vi "Make_RDDF_KBS.vi"() -> ()   [LabVIEW 2020]
uses:
  <vilib>/Utility/file.llb/Read Delimited Spreadsheet (DBL).vi
  <vilib>/Utility/file.llb/Write Delimited Spreadsheet (DBL).vi
panel:
  out "Y(long)":dbl format="%#_12g"
  out "X(lat)":dbl format="%#_12g"
  in  "stop":bool
  in  "file path (dialog if empty)":path caption="파일 경로(비었을 경우 대화 상자 창)"
  in  "dist.":dbl=0.2
  in  "?":bool
  out "XY 그래프":cluster{dbl[], dbl[]}[](graph)
  in  "File_Name(User):":string
  out "File_Name(Save):":string
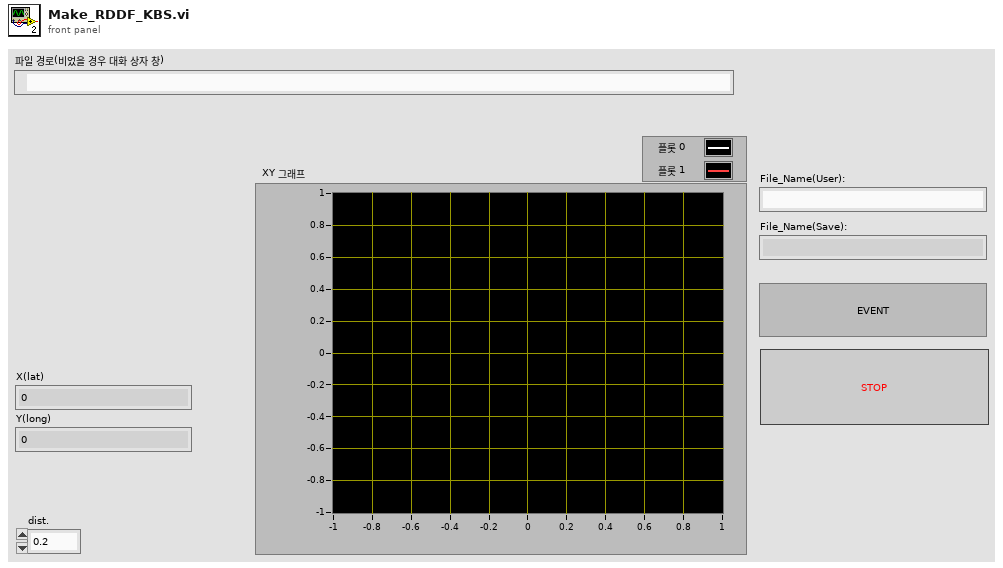
[diagram p1: front panel]
types:
  T1 = cluster{"X(lat)":dbl, "Y(long)":dbl, "Heading_T":dbl, "Heading_M":dbl, "GPS_SPD(kph)":dbl}
  T2 = enum16{"open", "replace", "create", "open or create", "replace or create", "replace or create with confirmation"}
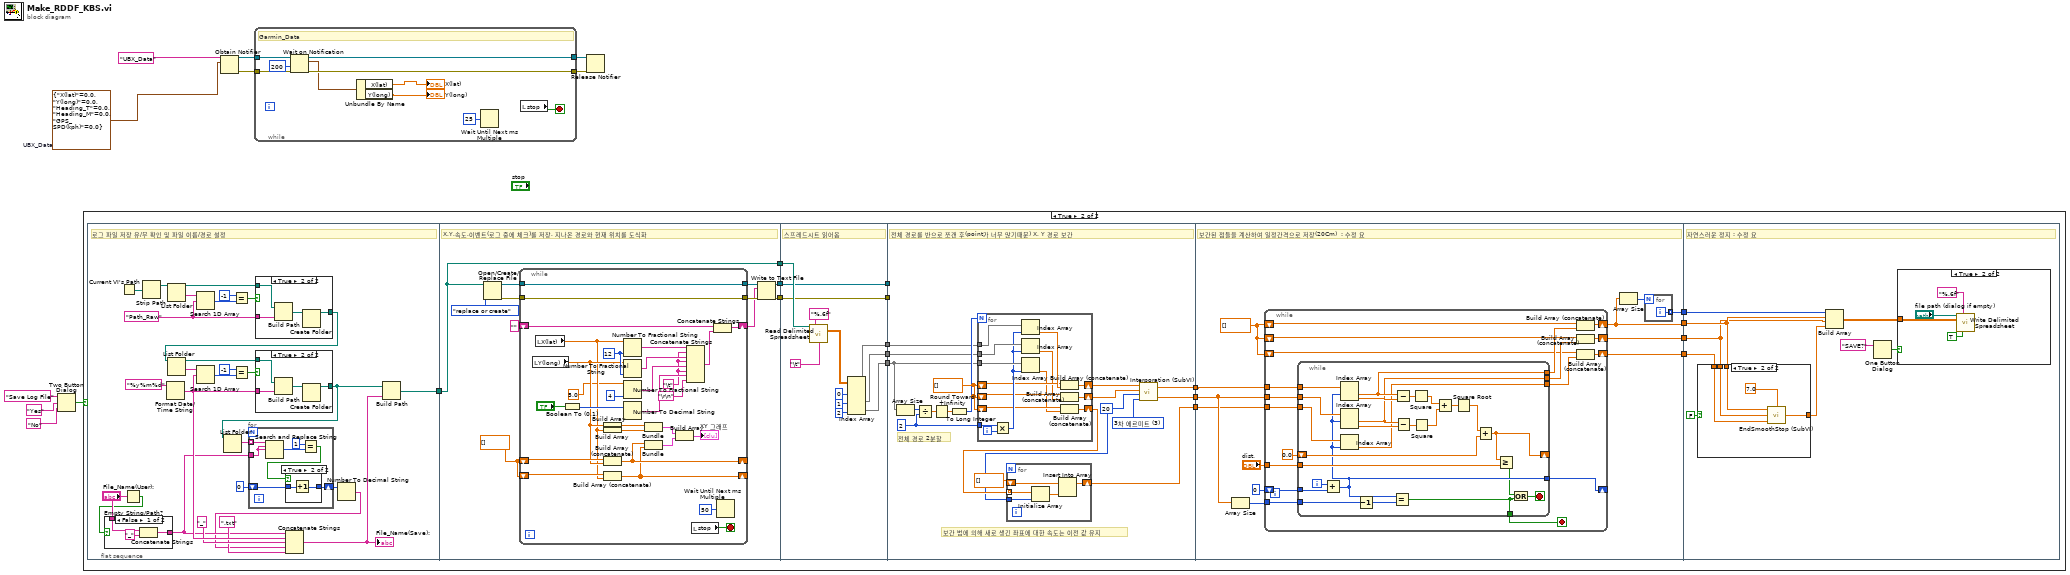
[diagram p0: block diagram]
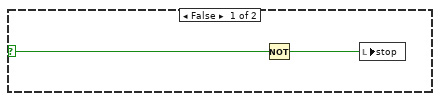
[diagram p2: hidden frame]
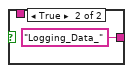
[diagram p3: hidden frame]
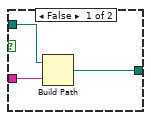
[diagram p5: hidden frame]
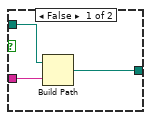
[diagram p6: hidden frame]
diagram:
  w1 = T1 {"X(lat)"=0.0, "Y(long)"=0.0, "Heading_T"=0.0, "Heading_M"=0.0, "GPS_SPD(kph)"=0.0}  # UBX_Data
  n1 = Two Button Dialog(message="Save Log File" ("메시지"), 1:"No" ("거짓 버튼 이름(\"취소\")"), 2:"Yes" ("참 버튼 이름(\"확인\")")) -> (T button?=w7:bool)
  n2 = case shown="True" w7 {
    selector: w7 -> [w12 _]
    frame False {
      n3 = Not(x=w12) -> (.not. x?=w11:bool)
      n4 = local write "stop"(w11) -> ()
    }
    frame True {
      n5 = flat-sequence {
        tunnel: [w56] -> w28
        tunnel: w28 -> [w88]
        tunnel: [w88] -> w27
        tunnel: [w87] -> w26
        tunnel: [w86] -> w25
        tunnel: w27 -> [w136]
        tunnel: w26 -> [w132]
        tunnel: w25 -> [w133]
        tunnel: [w133] -> w23
        tunnel: [w132] -> w22
        tunnel: [w125] -> w21
        tunnel: [w126] -> w20
        tunnel: [w130] -> w19
        tunnel: [w143] -> w24
        tunnel: w23 -> [_]
        tunnel: w22 -> [_]
        tunnel: w21 -> [w147]
        tunnel: w20 -> [w148]
        tunnel: w19 -> [w149]
        tunnel: [w138] -> w18
        tunnel: [w137] -> w17
        tunnel: w24 -> [w179]
        tunnel: w18 -> [w181]
        tunnel: w17 -> [w180]
        tunnel: [w178] -> w16
        tunnel: [w177] -> w15
        tunnel: [w176] -> w14
        tunnel: [w175] -> w13
        tunnel: w16 -> [w236]
        tunnel: w15 -> [w235]
        tunnel: w14 -> [w231]
        tunnel: w13 -> [w232]
        frame #0 {
          w51 = "Path_Raw" ("원소")
          # "로그 파일 저장 유/무 확인 및 파일 이름/경로 설정"
          n6 = Current VI's Path() -> (path=w55:path)
          n7 = Empty String/Path?(string/path="File_Name(User):") -> (empty?=w31:bool)
          n8 = case shown="False" w31 {
            tunnel: [w58 "Logging_Data_"] -> w35
            tunnel: "File_Name(User):" -> [w57 _]
            frame False {
              n9 = Concatenate Strings(w57, "_" ("문자열")) -> (w58:string)
            }
            frame True {
            }
          }
          n10 = Strip Path(path=w55) -> (stripped path=w54:path)  [unwired: 1 out]
          n11 = Format Date/Time String(time format string (%c)="%y%m%d" ("시간 포맷 문자열 (%c)")) -> (date/time string=w38:string)  [unwired: 2 in]
          n12 = List Folder(path=w54) -> (path out=w53:path, folder names=w50:string[])  [unwired: 3 in, 2 out]
          n13 = Search 1D Array(1D array=w50, element=w51) -> (index of element=w49:i32)  [unwired: 1 in]
          n14 = Equal?(x=-1 ("y"), y=w49) -> (x = y?=w52:bool)
          n15 = case shown="True" w52 {
            tunnel: w53 -> [w78 w83]
            tunnel: w51 -> [w79 w82]
            tunnel: [w80 w81] -> w41
            frame False {
              n16 = Build Path(base path=w78, name or relative path=w79) -> (appended path=w80:path)
            }
            frame True {
              n17 = Build Path(base path=w83, name or relative path=w82) -> (appended path=w84:path)
              n18 = Create Folder(path (use dialog)=w84) -> (created path=w81:path)  [unwired: 2 in, 2 out]
            }
          }
          n19 = List Folder(path=w41) -> (path out=w42:path, folder names=w44:string[])  [unwired: 3 in, 2 out]
          n20 = Search 1D Array(1D array=w44, element=w38) -> (index of element=w45:i32)  [unwired: 1 in]
          n21 = Equal?(x=-1 ("y"), y=w45) -> (x = y?=w43:bool)
          n22 = case shown="True" w43 {
            tunnel: w42 -> [w71 w76]
            tunnel: w38 -> [w72 w75]
            tunnel: [w73 w74] -> w30
            frame False {
              n23 = Build Path(base path=w71, name or relative path=w72) -> (appended path=w73:path)
            }
            frame True {
              n24 = Build Path(base path=w76, name or relative path=w75) -> (appended path=w77:path)
              n25 = Create Folder(path (use dialog)=w77) -> (created path=w74:path)  [unwired: 2 in, 2 out]
            }
          }
          n26 = List Folder(path=w30) -> (filenames=w40:string[])  [unwired: 3 in, 3 out]
          n27 = for {
            tunnel: w40 -> [w67] mode=indexing
            shift-right: [w62] -> w34
            shift-left: 0 -> [w63]
            tunnel: w35 -> [w61]
            n28 = Search and Replace String(input string=w67, search string=w61, replace string=w61) -> (number of replacements=w65:i32)  [unwired: 5 in, 3 out]
            n29 = Equal?(x=1, y=w65) -> (x = y?=w64:bool)
            n30 = case shown="True" w64 {
              tunnel: w63 -> [w68 w70]
              tunnel: [w68 w69] -> w62
              frame False {
              }
              frame True {
                n31 = Increment(x=w70) -> (x+1=w69:i32)
              }
            }
          }
          n32 = Number To Decimal String(number=w34) -> (decimal integer string=w33:string)  [unwired: 1 in]
          n33 = Concatenate Strings(w35, w38, "_" ("문자열"), w33, ".txt" ("문자열")) -> (w29:string)
          "File_Name(Save):" <- w29
          n34 = Build Path(base path=w30, name or relative path=w29) -> (appended path=w56:path)
        }
        frame #1 {
          w85 = dbl[] []
          # "X,Y,속도,이벤트(로그 중에 체크)를 저장, 지나온 경로와 현재 위치를 도식화"
          n35 = Open/Create/Replace File(file path (use dialog)=w88, operation (0:open)=T2."replace or create" ("동작(0:open)")) -> (refnum out=w93:refnum<file>, error out=w94:errorcluster)  [unwired: 4 in, 1 out]
          n36 = while {
            tunnel: w94 -> [w119]
            tunnel: w93 -> [w120]
            tunnel: [w120] -> w91
            tunnel: [w119] -> w92
            shift-right: [w104] -> w90
            shift-left: "" -> [w106]
            shift-right: [w100] -> _
            shift-left: w85 -> [w111]
            shift-right: [w99] -> _
            shift-left: w85 -> [w110]
            stop <- w118 stop-if-true
            w113 = "\t"
            w124 = i16 12 ("정밀도(6)")
            n37 = local read "Y(long)"() -> (w98:dbl)
            n38 = local read "X(lat)"() -> (w97:dbl)
            n39 = Boolean To (0,1)(Boolean="?") -> (0, 1=w121:i16)
            n40 = Build Array(w98) -> (w109:dbl[])
            n41 = Build Array(w97) -> (w108:dbl[])
            n42 = Build Array (concatenate)(w111, w98) -> (w100:dbl[])
            n43 = Build Array (concatenate)(w110, w97) -> (w99:dbl[])
            n44 = Number To Fractional String(number=w97, precision (6)=w124) -> (F-format string=w117:string)  [unwired: 2 in]
            n45 = Number To Fractional String(number=w98, precision (6)=w124) -> (F-format string=w116:string)  [unwired: 2 in]
            n46 = Number To Fractional String(number=5.0 ("x vel"), precision (6)=i16 4 ("정밀도(6)")) -> (F-format string=w115:string)  [unwired: 2 in]
            n47 = Number To Decimal String(number=w121) -> (decimal integer string=w114:string)  [unwired: 1 in]
            n48 = Bundle(w109, w108) -> (w101:cluster{dbl[], dbl[]})  [unwired: 1 in]
            n49 = Bundle(w100, w99) -> (w102:cluster{dbl[], dbl[]})  [unwired: 1 in]
            n50 = Build Array(w101, w102) -> (→"XY 그래프":cluster{dbl[], dbl[]}[])
            n51 = Concatenate Strings(w117, w113, w116, w113, w115, w113, w114, "\r\n") -> (w105:string)
            n52 = local read "stop"() -> (w118:bool)
            n53 = Concatenate Strings(w106, w105) -> (w104:string)
            n54 = Wait Until Next ms Multiple(millisecond multiple=u32 50 ("ms 배수")) -> ()  [unwired: 1 out]
          }
          n55 = Write to Text File(file (use dialog)=w91, text=w90, error in=w92) -> (refnum out=w86:refnum<file>, error out=w87:errorcluster)  [unwired: 1 in, 1 out]
        }
        frame #2 {
          # "스프레드시트 읽어옴"
          n56 = call-poly <vilib>:"Read Delimited Spreadsheet.vi"("file path (dialog if empty)"=w136, "format (%.3f)"="%.6f", "delimiter (\\t)"="\t") -> ("all rows"=w131:dbl[][])  [unwired: 7 in, 5 out]
          n57 = Index Array(array=w131, index (col) #1=0 ("비활성화된 인덱스 (열)"), index (col) #2=1 ("인덱스 (열)"), index (col) #3=2 ("인덱스 (열)")) -> (element #1=w130:dbl[], element #2=w126:dbl[], element #3=w125:dbl[])  [unwired: 3 in]
        }
        frame #3 {
          w142 = 3 items=["최근접", "선형", "스플라인", "3차 에르미트", "라그랑지"] ("method")
          w139 = 20 ("Interpolation factor (n)")
          w146 = dbl[] []
          w150 = 2
          # "보간 법에 의해 새로 생긴 좌표에 대한 속도는 이전 값 유지"
          # "전체 경로 2분할"
          # "전체 경로를 반으로 쪼갠 후(point가 너무 많기때문) X, Y 경로 보간"
          n58 = Array Size(array=w147) -> (size(s)=w154:i32)
          n59 = Divide(x=w154, y=w150) -> (x/y=w153:dbl)
          n60 = Round Toward +Infinity(x=w153) -> (ceil(x): smallest int >= x=w152:dbl)
          n61 = To Long Integer(number=w152) -> (32bit integer=w151:i32)
          n62 = for {
            N: w151 -> [_]
            tunnel: w150 -> [w173]
            tunnel: w149 -> [w172]
            tunnel: w148 -> [w171]
            tunnel: w147 -> [w170]
            shift-right: [w166] -> w141
            shift-left: w146 -> [w167]
            shift-right: [w165] -> w140
            shift-left: w146 -> [w163]
            shift-right: [w164] -> w145
            shift-left: w146 -> [w162]
            i -> [w174]
            n63 = Multiply(x=w173, y=w174) -> (x*y=w169:i32)
            n64 = Index Array(array=w172, index=w169) -> (element=w168:dbl)
            n65 = Index Array(array=w171, index=w169) -> (element=w161:dbl)
            n66 = Index Array(array=w170, index=w169) -> (element=w160:dbl)
            n67 = Build Array (concatenate)(w167, w168) -> (w166:dbl[])
            n68 = Build Array (concatenate)(w163, w161) -> (w165:dbl[])
            n69 = Build Array (concatenate)(w162, w160) -> (w164:dbl[])
          }
          n70 = for {
            tunnel: w145 -> [w159] mode=indexing
            tunnel: w139 -> [w158]
            shift-right: [w157] -> w143
            shift-left: dbl[] [] -> [w156]
            n71 = Initialize Array(w159, w158) -> (w155:dbl[])
            n72 = Insert Into Array(array=w156, new element=w155) -> (w157:dbl[])  [unwired: 1 in]
          }
          n73 = call "Interporation (SubVI).vi"("method"=w142, "Sample"=w139, "Y_long"=w140, "X_lat"=w141) -> ("Y_long"=w137:dbl[], "X_lat"=w138:dbl[])
        }
        frame #4 {
          w184 = dbl[] []
          # "보간된 점들을 계산하여 일정간격으로 저장(20Cm)  : 수정 요"
          n74 = Array Size(array=w180) -> (size(s)=w183:i32)
          n75 = while {
            tunnel: "dist." -> [w202]
            tunnel: w181 -> [w205]
            tunnel: w180 -> [w204]
            tunnel: w179 -> [w196]
            shift-right: [w191] -> _
            shift-left: 0 -> [w201]
            shift-right: [w188] -> w175
            shift-left: w184 -> [w197]
            shift-right: [w190] -> w176
            shift-left: w184 -> [w198]
            shift-right: [w189] -> w177
            shift-left: w184 -> [w194]
            tunnel: w183 -> [w193]
            stop <- w192 stop-if-true
            n76 = while {
              tunnel: w205 -> [w230]
              tunnel: w204 -> [w229]
              shift-right: [w219] -> _
              shift-left: 0.0 -> [w220]
              tunnel: w202 -> [w218]
              tunnel: [w210] -> w191
              tunnel: w201 -> [w216]
              tunnel: [w215] -> w200
              tunnel: [w214] -> w199
              tunnel: w196 -> [w213]
              tunnel: [w212] -> w195
              tunnel: w193 -> [w211]
              tunnel: [w207] -> w192
              i -> [w217]
              stop <- w209 stop-if-true
              n77 = Add(x=w217, y=w216) -> (x+y=w210:i32)
              n78 = Index Array(array=w230, index #1=w210) -> (element #1=w215:dbl, element #2=w228:dbl)  [unwired: 1 in]
              n79 = Index Array(array=w229, index #1=w210) -> (element #1=w214:dbl, element #2=w227:dbl)  [unwired: 1 in]
              n80 = Index Array(array=w213, index=w210) -> (element=w212:dbl)
              n81 = Decrement(x=w211) -> (x-1=w206:i32)
              n82 = Equal?(x=w210, y=w206) -> (x = y?=w207:bool)
              n83 = Subtract(x=w215, y=w228) -> (x-y=w226:dbl)
              n84 = Subtract(x=w214, y=w227) -> (x-y=w225:dbl)
              n85 = Square(x=w226) -> (x^2=w224:dbl)
              n86 = Square(x=w225) -> (x^2=w223:dbl)
              n87 = Add(x=w224, y=w223) -> (x+y=w222:dbl)
              n88 = Square Root(x=w222) -> (sqrt(x)=w221:dbl)
              n89 = Add(x=w221, y=w220) -> (x+y=w219:dbl)
              n90 = Greater Or Equal?(x=w219, y=w218) -> (x >= y?=w208:bool)
              n91 = Or(x=w208, y=w207) -> (x .or. y?=w209:bool)
            }
            n92 = Build Array (concatenate)(w197, w200) -> (w188:dbl[])
            n93 = Build Array (concatenate)(w198, w199) -> (w190:dbl[])
            n94 = Build Array (concatenate)(w194, w195) -> (w189:dbl[])
          }
          n95 = Array Size(array=w175) -> (size(s)=w182:i32)
          n96 = for {
            N: w182 -> [_]
            tunnel: [w187] -> w178 mode=indexing
            i -> [w187]
          }
        }
        frame #5 {
          # "자연스러운 정지 : 수정 요"
          n97 = case shown="True" FALSE {
            tunnel: w232 -> [_ w245]
            tunnel: w231 -> [_ w244]
            tunnel: w235 -> [w240 w243]
            tunnel: [w240 w241] -> w238
            frame False {
            }
            frame True {
              n98 = call "EndSmoothStop (SubVI).vi"("meter"=7.0, "V_arr"=w243, "Y_arr"=w244, "X_arr"=w245) -> ("V_arr_new"=w241:dbl[])
            }
          }
          n99 = Build Array(w236, w232, w231, w238) -> (w239:dbl[][])
          n100 = One Button Dialog(message="SAVE?") -> (true=w234:bool)  [unwired: 1 in]
          n101 = case shown="True" w234 {
            tunnel: w239 -> [_ w249]
            frame False {
            }
            frame True {
              n102 = call-poly <vilib>:"Write Delimited Spreadsheet.vi"("file path (dialog if empty)"="file path (dialog if empty)", "format (%.3f)"="%.6f", "2D data"=w249, "transpose? (no:F)"=TRUE) -> ()  [unwired: 10 in, 2 out]
            }
          }
        }
      }
    }
  }
  n103 = Obtain Notifier(name (unnamed)="UBX_Data" ("이름(이름없음)"), notification data type=w1) -> (notifier out=w5:refnum<notifier>, error out=w6:errorcluster)  [unwired: 2 in, 1 out]
  n104 = while {
    tunnel: w5 -> [w259]
    tunnel: w6 -> [w258]
    tunnel: [w257] -> w3
    tunnel: [w256] -> w4
    stop <- w250 stop-if-true
    # "Garmin_Data"
    n105 = Wait on Notification(notifier=w259, timeout in ms (-1)=200 ("타임아웃(ms) (-1)"), error in (no error)=w258) -> (notifier out=w257:refnum<notifier>, notification=w255:T1, error out=w256:errorcluster)  [unwired: 1 in, 1 out]
    n106 = Unbundle By Name(w255) -> ("X(lat)"=→"X(lat)":dbl, "Y(long)"=→"Y(long)":dbl)
    n107 = Wait Until Next ms Multiple(millisecond multiple=u32 25) -> ()  [unwired: 1 out]
    n108 = local read "stop"() -> (w250:bool)
  }
  n109 = Release Notifier(notifier=w3, error in (no error)=w4) -> ()  [unwired: 1 in, 3 out]
